vi "CommSelector.vi"(0 "VISA resource name":refnum<visa-resource-name>) -> (4 "VISA resource name":refnum<visa-resource-name>, 8 "CommType":string)   [LabVIEW 2011]
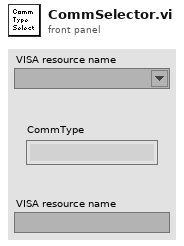
[diagram p1: front panel]
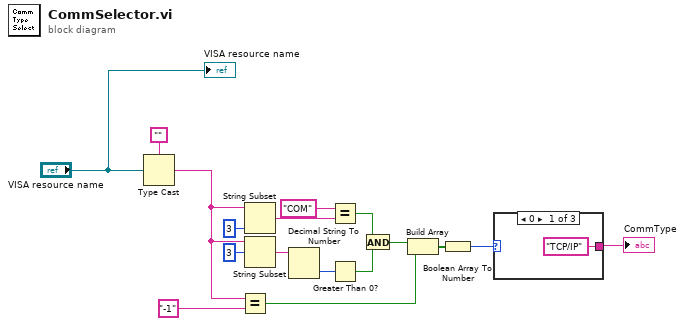
[diagram p0: block diagram]
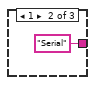
[diagram p2: hidden frame]
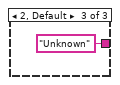
[diagram p3: hidden frame]
diagram:
  n1 = Type Cast(type="", x="VISA resource name") -> (*(type *) &x=w15:string)
  n2 = Equal?(x=w15, y="-1") -> (x = y?=w6:bool)
  n3 = String Subset(string=w15, length (rest)=3 ("length (rest)")) -> (substring=w12:string)  [unwired: 1 in]
  n4 = String Subset(string=w15, offset (0)=3) -> (substring=w10:string)  [unwired: 1 in]
  n5 = Decimal String To Number(string=w10) -> (number=w9:i32)  [unwired: 2 in, 1 out]
  n6 = Equal?(x="COM", y=w12) -> (x = y?=w8:bool)
  n7 = Greater Than 0?(x=w9) -> (x > 0?=w7:bool)
  n8 = And(x=w8, y=w7) -> (x .and. y?=w5:bool)
  n9 = Build Array(w5, w6) -> (w4:bool[])
  n10 = Boolean Array To Number(Boolean array=w4) -> (number=w3:u32)
  n11 = case shown="0" w3 {
    tunnel: ["TCP/IP" ("x") "Serial" ("x") "Unknown" ("x")] -> w2
    frame 0 {
    }
    frame 1 {
    }
    frame 2, Default {
    }
  }
  "CommType" <- w2
  "VISA resource name" <- "VISA resource name"
